vi "Teleop.vi"(10 "Match Info":T1={"Autonomous Elapsed Seconds"=0.0, "TeleOp Elapsed Seconds"=0.0, "Disabled Elapsed Seconds"=0.0, "Visited Autonomous"=FALSE, "Visited TeleOp"=FALSE, "Visited Disabled"=FALSE, "Autonomous Settings"={"Autonomous Style"=enum."Independent", "VI Refnum"=refnum}}, 11 "Call Context":T2) -> ()   [LabVIEW 2016]
doc: "This VI is called for each TeleOp packet received from the DS where the robot is not disabled. It is often used to read from the joysticks and update I/O or to update setpoints for timed control loops. It should complete and return within 20 milliseconds or it may miss DS packets."
uses:
  <vilib>/Rock Robotics/WPI/DriverStation/WPI_DriverStationDerivedRobotMode.ctl
  <vilib>/Rock Robotics/WPI/DriverStation/WPI_DriverStationMatch Info.ctl
  <vilib>/Rock Robotics/WPI/Utilities/WPI_GetSetVariantRefNum.vi
  <vilib>/Rock Robotics/Network Tables/NT Write Boolean Array.vi
  <vilib>/Rock Robotics/Network Tables/NT Write Numeric Array.vi
  <vilib>/Rock Robotics/Network Tables/NT Read Boolean.vi
  <vilib>/Rock Robotics/Network Tables/NT Write Number.vi
  <vilib>/Rock Robotics/Network Tables/NT Write Boolean.vi
  <vilib>/Rock Robotics/Network Tables/NT Read Number.vi
panel:
  out "Limit?":bool
  out "Lift Bottom":dbl
  out "Lift Top":dbl
  out "Sample Boolean 1":bool
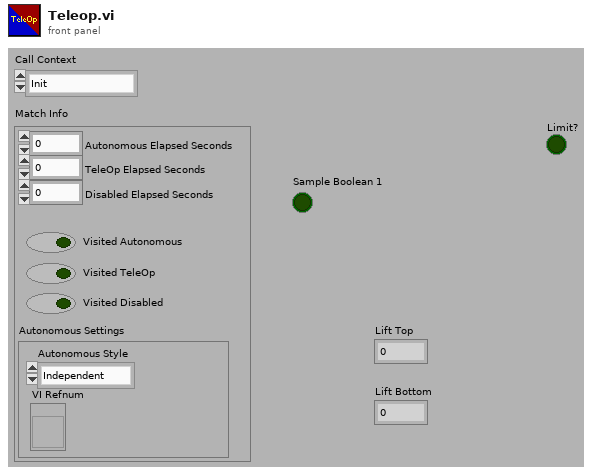
[diagram p1: front panel]
types:
  T1 = typedef "WPI_DriverStationMatch Info.ctl" = cluster{"Autonomous Elapsed Seconds":dbl, "TeleOp Elapsed Seconds":dbl, "Disabled Elapsed Seconds":dbl, "Visited Autonomous":bool, "Visited TeleOp":bool, "Visited Disabled":bool, "Autonomous Settings":cluster{"Autonomous Style":enum16{"Iterative", "Independent"}, "VI Refnum":refnum<vi>}}
  T2 = typedef "WPI_DriverStationDerivedRobotMode.ctl" = enum16{"Init", "Execute", "Stop"}
  T3 = typedef "WPI_GyroDevRef.ctl" = cluster{"DevStatus":errorcluster, "Analog Channel":T4, "Offset":dbl, "Gain (VoltsPerDegree/Second)":dbl, "Gyro Type":enum16{"Analog", "XRS450"}, "Handle":i32, "SPI Bus":T5, "Device Found":bool, "Sample Rate":dbl, "Calibrate On Open":bool}
  T4 = typedef "FPGA_AIChannel.ctl" = enum8{"AI 0", "AI 1", "AI 2", "AI 3", "AI MXP 0", "AI MXP 1", "AI MXP 2", "AI MXP 3", "Invalid"}
  T5 = typedef "spi_bus.ctl" = enum16{"SPI On-Board, CS0", "SPI On-Board, CS1", "SPI On-Board, CS2", "SPI On-Board, CS3", "SPI MXP", "Invalid"}
  T6 = typedef "WPI_JoystickDevRef.ctl" = cluster{"Device":T7}
  T7 = typedef "WPI_JoystickDeviceEnum.ctl" = enum16{"USB 0", "USB 1", "USB 2", "USB 3", "USB 4", "USB 5"}
  T8 = cluster{"Buttons[0]":bool, "Buttons[1]":bool, "Buttons[2]":bool, "Buttons[3]":bool, "Buttons[4]":bool, "Buttons[5]":bool, "Buttons[6]":bool, "Buttons[7]":bool, "Buttons[8]":bool}
  T9 = typedef "WPI_RobotDriveDevRef.ctl" = cluster{"DevStatus":errorcluster, "Motors[]":T10[], "Square Inputs":bool, "Max Output":dbl}
  T10 = typedef "WPI_MotorControlDeviceRef.ctl" = cluster{"DeviceStatus":errorcluster, "Type":T11, "PWM":cluster{"PWM Channel":T12, "DeadBand":T13}, "CAN":cluster{"Device Number":u8, "SetOutput VI Ref":variant, "GetOutput VI Ref":variant, "Enable VI Ref":variant, "Disable VI Ref":variant, "Data":variant}, "Invert":bool}
  T11 = typedef "WPI_MotorControlType.ctl" = enum16{"PWM", "CAN"}
  T12 = typedef "FPGA_DIOPWMChannel.ctl" = enum8{"PWM 0", "PWM 1", "PWM 2", "PWM 3", "PWM 4", "PWM 5", "PWM 6", "PWM 7", "PWM 8", "PWM 9", "PWM MXP 0", "PWM MXP 1", "PWM MXP 2", "PWM MXP 3", "PWM MXP 4", "PWM MXP 5", "PWM MXP 6", "PWM MXP 7", "PWM MXP 8", "PWM MXP 9", "Invalid"}
  T13 = typedef "WPI_PWMDeadband.ctl" = cluster{"Name":string, "maxPositivePwm":i32, "minPositivePwm":i32, "centerPwm":i32, "maxNegativePwm":i32, "minNegativePwm":i32, "angularRange":u16}
  T14 = cluster{"Axes[0]":dbl, "Axes[1]":dbl, "Axes[2]":dbl, "Axes[3]":dbl, "Axes[4]":dbl, "Axes[5]":dbl, "Axes[6]":dbl, "Axes[7]":dbl, "Axes[8]":dbl}
  T15 = typedef "WPI_DigitalInputDevRef.ctl" = cluster{"DevStatus":errorcluster, "DIO Channel":T16}
  T16 = typedef "FPGA_DIOChannel.ctl" = enum8{"DIO 0", "DIO 1", "DIO 2", "DIO 3", "DIO 4", "DIO 5", "DIO 6", "DIO 7", "DIO 8", "DIO 9", "DIO MXP 0", "DIO MXP 1", "DIO MXP 2", "DIO MXP 3", "DIO MXP 4", "DIO MXP 5", "DIO MXP 6", "DIO MXP 7", "DIO MXP 8", "DIO MXP 9", "DIO MXP 10", "DIO MXP 11", "DIO MXP 12", "DIO MXP 13", "DIO MXP 14", "DIO MXP 15", "SPI Port CS1", "SPI Port CS2", "SPI Port CS3", "SPI Port MISO", "SPI Port MOSI", "Invalid"}
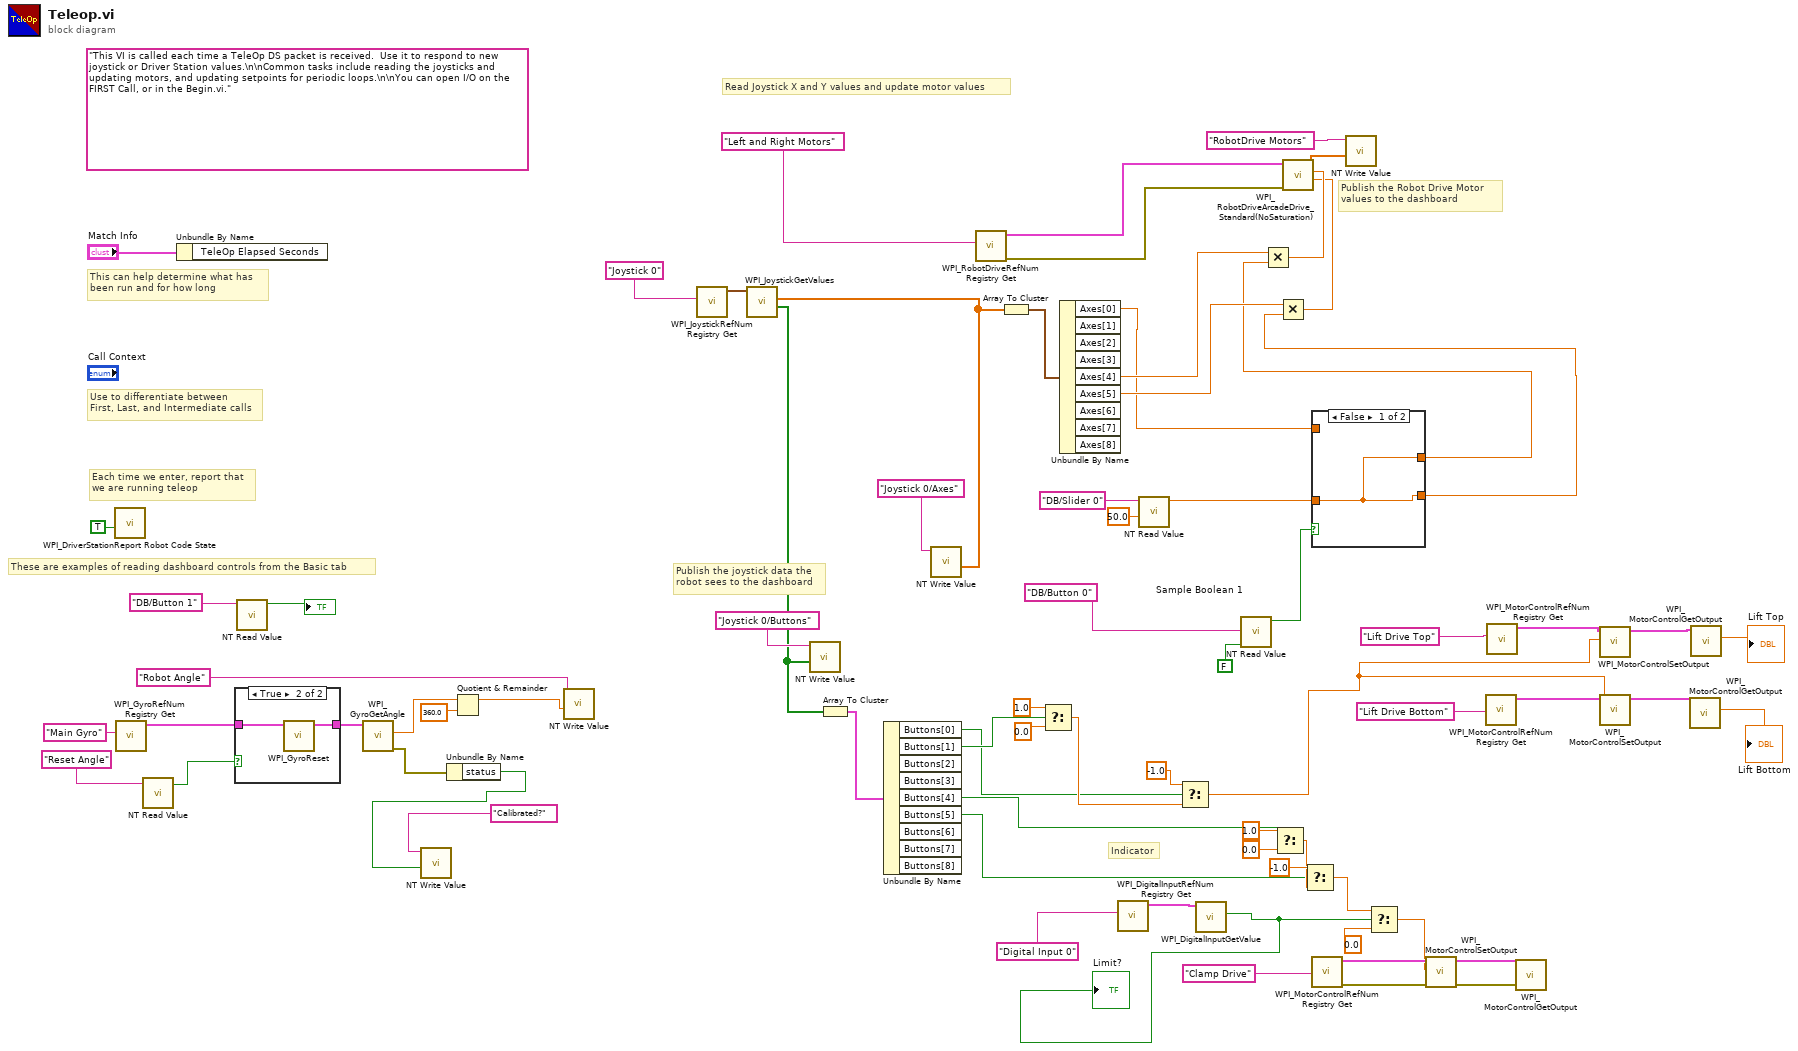
[diagram p0: block diagram]
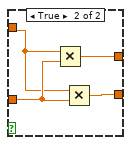
[diagram p2: hidden frame]
diagram:
  (unwired) "This VI is called each time a TeleOp DS packet is received.  Use it to respond to new joystick or Driver Station values.\n\nCommon tasks include reading the joysticks and updating motors, and updating setpoints for periodic loops.\n\nYou can open I/O on the FIRST Call, or in the Begin.vi."
  # "Indicator"
  # "These are examples of reading dashboard controls from the Basic tab"
  # "Publish the Robot Drive Motor\nvalues to the dashboard"
  # "Publish the joystick data the\nrobot sees to the dashboard"
  # "Each time we enter, report that\nwe are running teleop"
  # "Use to differentiate between\nFirst, Last, and Intermediate calls"
  # "This can help determine what has\nbeen run and for how long"
  # "Read Joystick X and Y values and update motor values"
  n1 = call <vilib>:"WPI_DriverStationReport Robot Code State.vi"("TeleOp"=TRUE ("Autonomous")) -> ()  [unwired: 10 in, 1 out]
  n2 = call <vilib>:"WPI_GyroRefNum Registry Get.vi"("refnum name"="Main Gyro") -> ("GyroDevRef"=w27:T3)  [unwired: 9 in, 1 out]
  n3 = call-poly <vilib>:"NT Read Value.vi"("Name"="Reset Angle") -> ("Boolean"=w24:bool)  [unwired: 9 in, 1 out]
  n4 = Unbundle By Name("Match Info") -> ()  [unwired: 1 out]
  n5 = case shown="True" w24 {
    tunnel: [w75 w77] -> w31
    tunnel: w27 -> [w75 w76]
    frame False {
    }
    frame True {
      n6 = call <vilib>:"WPI_GyroReset.vi"("GyroDevRef"=w76) -> ("GyroDevRef"=w77:T3)  [unwired: 9 in, 1 out]
    }
  }
  n7 = call-poly <vilib>:"NT Read Value.vi"("Name"="DB/Button 1" ("refnum name")) -> ("Boolean"=→"Sample Boolean 1":bool)  [unwired: 9 in, 1 out]
  n8 = call <vilib>:"WPI_GyroGetAngle.vi"("GyroDevRef"=w31) -> ("error out"=w29:errorcluster, "Angle"=w30:dbl)  [unwired: 7 in, 2 out]
  n9 = Unbundle By Name(w29) -> ("status"=w2:bool)
  n10 = call-poly <vilib>:"NT Write Value.vi"("Boolean"=w2, "Name"="Calibrated?") -> ()  [unwired: 9 in, 1 out]
  n11 = Quotient & Remainder(x=w30, y=360.0) -> (x-y*floor(x/y)=w26:dbl)  [unwired: 1 out]
  n12 = call-poly <vilib>:"NT Write Value.vi"("Numeric"=w26, "Name"="Robot Angle") -> ()  [unwired: 9 in, 1 out]
  n13 = call <vilib>:"WPI_JoystickRefNum Registry Get.vi"("refnum name"="Joystick 0") -> ("JoystickDevRef"=w71:T6)  [unwired: 1 in, 9 out]
  n14 = call <vilib>:"WPI_JoystickGetValues.vi"("JoystickDevRef"=w71) -> ("Buttons"=w4:bool[], "Axes"=w17:dbl[])  [unwired: 6 in, 3 out]
  n15 = call-poly <vilib>:"NT Write Value.vi"("Boolean Array"=w4, "Name"="Joystick 0/Buttons") -> ()  [unwired: 9 in, 1 out]
  n16 = Array To Cluster(array=w4) -> (cluster=w18:T8)
  n17 = Unbundle By Name(w18) -> ("Buttons[0]"=w3:bool, "Buttons[1]"=w21:bool, "Buttons[4]"=w20:bool, "Buttons[5]"=w19:bool)  [unwired: 5 out]
  n18 = call-poly <vilib>:"NT Write Value.vi"("Numeric Array"=w17, "Name"="Joystick 0/Axes") -> ()  [unwired: 9 in, 1 out]
  n19 = call <vilib>:"WPI_RobotDriveRefNum Registry Get.vi"("refnum name"="Left and Right Motors") -> ("error out"=w13:errorcluster, "RobotDriveDevRef"=w72:T9)  [unwired: 1 in, 8 out]
  n20 = Array To Cluster(array=w17) -> (cluster=w16:T14)
  n21 = Select(t=1.0, s=w21, f=0.0) -> (s? t:f=w47:dbl)
  n22 = Unbundle By Name(w16) -> ("Axes[0]"=w6:dbl, "Axes[4]"=w15:dbl, "Axes[5]"=w14:dbl)  [unwired: 6 out]
  n23 = call <vilib>:"WPI_DigitalInputRefNum Registry Get.vi"("refnum name"="Digital Input 0") -> ("DigitalInputDevRef"=w36:T15)  [unwired: 9 in, 1 out]
  n24 = call-poly <vilib>:"NT Read Value.vi"("Default Value"=50.0, "Name"="DB/Slider 0" ("refnum name")) -> ("Numeric"=w7:dbl)  [unwired: 8 in, 1 out]
  n25 = Select(t=-1.0, s=w3, f=w47) -> (s? t:f=w48:dbl)
  n26 = call <vilib>:"WPI_DigitalInputGetValue.vi"("DigitalInputDevRef"=w36) -> ("Value"=w1:bool)  [unwired: 8 in, 2 out]
  "Limit?" <- w1
  n27 = call-poly <vilib>:"NT Read Value.vi"("Default Value"=FALSE, "Name"="DB/Button 0" ("refnum name")) -> ("Boolean"=w11:bool)  [unwired: 8 in, 1 out]
  n28 = Select(t=1.0, s=w20, f=0.0) -> (s? t:f=w38:dbl)
  n29 = Select(t=-1.0, s=w19, f=w38) -> (s? t:f=w35:dbl)
  n30 = case shown="False" w11 {
    tunnel: w6 -> [_ w79]
    tunnel: [w78 w82] -> w8
    tunnel: [w78 w81] -> w9
    tunnel: w7 -> [w78 w80]
    frame False {
    }
    frame True {
      n31 = Multiply(x=w79, y=w80) -> (x*y=w82:dbl)
      n32 = Multiply(x=w79, y=w80) -> (x*y=w81:dbl)
    }
  }
  n33 = Multiply(x=w15, y=w8) -> (x*y=w61:dbl)
  n34 = Multiply(x=w14, y=w9) -> (x*y=w60:dbl)
  n35 = call <vilib>:"WPI_RobotDriveArcadeDrive_Standard(NoSaturation).vi"("error in (no error)"=w13, "Y axis value"=w60, "X axis value"=w61, "RobotDriveDevRef"=w72) -> ("Motor Values"=w64:dbl[])  [unwired: 7 out]
  n36 = call <vilib>:"WPI_MotorControlRefNum Registry Get.vi"("refnum name"="Clamp Drive") -> ("error out"=w46:errorcluster, "MotorControlDevRef"=w44:T10)  [unwired: 9 in]
  n37 = call-poly <vilib>:"NT Write Value.vi"("Numeric Array"=w64, "Name"="RobotDrive Motors") -> ()  [unwired: 9 in, 1 out]
  n38 = Select(t=w35, s=w1, f=0.0) -> (s? t:f=w34:dbl)
  n39 = call <vilib>:"WPI_MotorControlSetOutput.vi"("error in (no error)"=w46, "Output"=w34, "MotorControlDevRef"=w44) -> ("error out"=w43:errorcluster, "MotorControlDevRef"=w45:T10)  [unwired: 6 in, 1 out]
  n40 = call <vilib>:"WPI_MotorControlRefNum Registry Get.vi"("refnum name"="Lift Drive Bottom") -> ("MotorControlDevRef"=w56:T10)  [unwired: 9 in, 1 out]
  n41 = call <vilib>:"WPI_MotorControlRefNum Registry Get.vi"("refnum name"="Lift Drive Top") -> ("MotorControlDevRef"=w57:T10)  [unwired: 9 in, 1 out]
  n42 = call <vilib>:"WPI_MotorControlGetOutput.vi"("error in (no error)"=w43, "MotorControlDevRef"=w45) -> ()  [unwired: 7 in, 3 out]
  n43 = call <vilib>:"WPI_MotorControlSetOutput.vi"("Output"=w48, "MotorControlDevRef"=w57) -> ("MotorControlDevRef"=w58:T10)  [unwired: 7 in, 2 out]
  n44 = call <vilib>:"WPI_MotorControlSetOutput.vi"("Output"=w48, "MotorControlDevRef"=w56) -> ("MotorControlDevRef"=w59:T10)  [unwired: 7 in, 2 out]
  n45 = call <vilib>:"WPI_MotorControlGetOutput.vi"("MotorControlDevRef"=w59) -> ("Output"=→"Lift Bottom":dbl)  [unwired: 8 in, 2 out]
  n46 = call <vilib>:"WPI_MotorControlGetOutput.vi"("MotorControlDevRef"=w58) -> ("Output"=→"Lift Top":dbl)  [unwired: 8 in, 2 out]
